vi "initalize 6221-2182-dc(SubVI).vi"(9 "字符串":string, 11 "簇":T13={"initialize"=enum."SR830", "6221"={"6221 Resource"="GPIB0::24::INSTR", "Delta status"=FALSE, "电流|RMS(A)"=0.0}, "SR830+6221"={"source"=0, "Current(A)"=0.0, "阻抗(Ohm)"=0.0, "SR830 1"=FALSE, "SR830 2"=FALSE, "SR830 3"=FALSE, "SR830 4"=FALSE, "VISA 1"="", "VISA 2"="", "VISA 3"="", "VISA 4"="", "Reserve 1"=0, "Reserve 2"=-1, "Reserve 3"=-1, "Reserve 4"=-1, "Sensitivity 1"=-1, "Sensitivity 2"=0, "Sensitivity 3"=-1, "Sensitivity 4"=-1, "量程入 1"=0, "量程入 2"=0, "量程入 3"=0, "量程入 4"=0}, "2400"={"2400"=FALSE, "VISA"="", "Output Level (0)"=1e-05, "Compliance  Level (0.1)"=10.0}, "ch"={"ch"=[], "current"=[], "change?"=[], "holding current\nwhen change ch?"=FALSE}, "Instrument"={"335 Resource"="GPIB0::24::INSTR", "Input (0:A)"=0, "Instrument Type"=enum."PPMS-Rotate", "quantum design"=refnum, "Heater Output (1:1)"=1, "semaphore"=refnum, "TCP master instance"=refnum, "335 Status"=refnum, "M24C Resource"="GPIB0::24::INSTR", "4G supply"="GPIB0::24::INSTR", "Temp Status 24C"=refnum, "Temp"=refnum, "9T信号"=refnum, "limit"={"Field limit"=0.0, "Field rate limit"=0.0, "Temp limit"=0.0, "Temp low limit"=0.0, "Temp rate limit "=0.0}, "4g supply status"=refnum, "vi路径"="", "325 Resource "="GPIB0::24::INSTR", "Input (0:A) 325"=0, "Input (1;B)"=1, "in-plane"="", "out-plane"="", "in-plane"=FALSE, "out-plane"=FALSE}, "Aborting"=refnum, "数据文件"=refnum, "warning"=refnum, "2614B"={"2614B chA"=FALSE, "2614B chB"=FALSE, "VISA"=""}, "33522b"={"33522b resource name"="", "零电压"=0.0, "最大电压"=148.0, "间隔"=4.0, "最小电压"=-48.0, "PZT Scan?"=FALSE}, "gating type"=enum."2614(daul)"} {"Instrument"."Input (1;B)" items=["A", "B"]; "Instrument"."Input (0:A) 325" items=["A", "B"]; "Instrument"."Input (0:A)" items=["A", "B"]; "Instrument"."Heater Output (1:1)" items=["1"=1, "2"=2]; "SR830+6221"."Sensitivity 4" items=["Auto Gain"=-1, "2 nV/fA"=0, "5 nV/fA"=1, "10 nV/fA"=2, "20 nV/fA"=3, "50 nV/fA"=4, "100 nV/fA"=5, "200 nV/fA"=6, "500 nV/fA"=7, "1 uV/pA"=8, "2 uV/pA"=9, "5 uV/pA"=10, "10 uV/pA"=11, "20 uV/pA"=12, "50 uV/pA"=13, "100 uV/pA"=14, "200 uV/pA"=15, "500 uV/pA"=16, "1 mV/nA"=17, "2 mV/nA"=18, "5 mV/nA"=19, "10 mV/nA"=20, "20 mV/nA"=21, "50 mV/nA"=22, "100 mV/nA"=23, "200 mV/nA"=24, "500 mV/mA"=25, "1 V/uA"=26]; "SR830+6221"."Sensitivity 3" items=["Auto Gain"=-1, "2 nV/fA"=0, "5 nV/fA"=1, "10 nV/fA"=2, "20 nV/fA"=3, "50 nV/fA"=4, "100 nV/fA"=5, "200 nV/fA"=6, "500 nV/fA"=7, "1 uV/pA"=8, "2 uV/pA"=9, "5 uV/pA"=10, "10 uV/pA"=11, "20 uV/pA"=12, "50 uV/pA"=13, "100 uV/pA"=14, "200 uV/pA"=15, "500 uV/pA"=16, "1 mV/nA"=17, "2 mV/nA"=18, "5 mV/nA"=19, "10 mV/nA"=20, "20 mV/nA"=21, "50 mV/nA"=22, "100 mV/nA"=23, "200 mV/nA"=24, "500 mV/mA"=25, "1 V/uA"=26]; "SR830+6221"."Sensitivity 1" items=["Auto Gain"=-1, "2 nV/fA"=0, "5 nV/fA"=1, "10 nV/fA"=2, "20 nV/fA"=3, "50 nV/fA"=4, "100 nV/fA"=5, "200 nV/fA"=6, "500 nV/fA"=7, "1 uV/pA"=8, "2 uV/pA"=9, "5 uV/pA"=10, "10 uV/pA"=11, "20 uV/pA"=12, "50 uV/pA"=13, "100 uV/pA"=14, "200 uV/pA"=15, "500 uV/pA"=16, "1 mV/nA"=17, "2 mV/nA"=18, "5 mV/nA"=19, "10 mV/nA"=20, "20 mV/nA"=21, "50 mV/nA"=22, "100 mV/nA"=23, "200 mV/nA"=24, "500 mV/mA"=25, "1 V/uA"=26]; "SR830+6221"."Sensitivity 2" items=["Auto Gain"=-1, "2 nV/fA"=0, "5 nV/fA"=1, "10 nV/fA"=2, "20 nV/fA"=3, "50 nV/fA"=4, "100 nV/fA"=5, "200 nV/fA"=6, "500 nV/fA"=7, "1 uV/pA"=8, "2 uV/pA"=9, "5 uV/pA"=10, "10 uV/pA"=11, "20 uV/pA"=12, "50 uV/pA"=13, "100 uV/pA"=14, "200 uV/pA"=15, "500 uV/pA"=16, "1 mV/nA"=17, "2 mV/nA"=18, "5 mV/nA"=19, "10 mV/nA"=20, "20 mV/nA"=21, "50 mV/nA"=22, "100 mV/nA"=23, "200 mV/nA"=24, "500 mV/mA"=25, "1 V/uA"=26]; "SR830+6221"."Reserve 4" items=["Auto Gain"=-1, "2 nV/fA"=0, "5 nV/fA"=1, "10 nV/fA"=2, "20 nV/fA"=3, "50 nV/fA"=4, "100 nV/fA"=5, "200 nV/fA"=6, "500 nV/fA"=7, "1 uV/pA"=8, "2 uV/pA"=9, "5 uV/pA"=10, "10 uV/pA"=11, "20 uV/pA"=12, "50 uV/pA"=13, "100 uV/pA"=14, "200 uV/pA"=15, "500 uV/pA"=16, "1 mV/nA"=17, "2 mV/nA"=18, "5 mV/nA"=19, "10 mV/nA"=20, "20 mV/nA"=21, "50 mV/nA"=22, "100 mV/nA"=23, "200 mV/nA"=24, "500 mV/mA"=25, "1 V/uA"=26]; "SR830+6221"."Reserve 3" items=["Auto Reserve"=-1, "High Reserve"=0, "Normal"=1, "Low Noise"=2]; "SR830+6221"."Reserve 2" items=["Auto Reserve"=-1, "High Reserve"=0, "Normal"=1, "Low Noise"=2]; "SR830+6221"."Reserve 1" items=["Auto Reserve"=-1, "High Reserve"=0, "Normal"=1, "Low Noise"=2]; "SR830+6221"."source" items=["SR830 1", "SR830 2", "SR830 3", "SR830 4"]}) -> (3 "输出簇":T13={"initialize"=enum."SR830", "6221"={"6221 Resource"="GPIB0::24::INSTR", "Delta status"=FALSE, "电流|RMS(A)"=0.0}, "SR830+6221"={"source"=0, "Current(A)"=0.0, "阻抗(Ohm)"=0.0, "SR830 1"=FALSE, "SR830 2"=FALSE, "SR830 3"=FALSE, "SR830 4"=FALSE, "VISA 1"="", "VISA 2"="", "VISA 3"="", "VISA 4"="", "Reserve 1"=0, "Reserve 2"=-1, "Reserve 3"=-1, "Reserve 4"=-1, "Sensitivity 1"=-1, "Sensitivity 2"=0, "Sensitivity 3"=-1, "Sensitivity 4"=-1, "量程入 1"=0, "量程入 2"=0, "量程入 3"=0, "量程入 4"=0}, "2400"={"2400"=FALSE, "VISA"="", "Output Level (0)"=1e-05, "Compliance  Level (0.1)"=10.0}, "ch"={"ch"=[], "current"=[], "change?"=[], "holding current\nwhen change ch?"=FALSE}, "Instrument"={"335 Resource"="GPIB0::24::INSTR", "Input (0:A)"=0, "Instrument Type"=enum."PPMS-Rotate", "quantum design"=refnum, "Heater Output (1:1)"=1, "semaphore"=refnum, "TCP master instance"=refnum, "335 Status"=refnum, "M24C Resource"="GPIB0::24::INSTR", "4G supply"="GPIB0::24::INSTR", "Temp Status 24C"=refnum, "Temp"=refnum, "9T信号"=refnum, "limit"={"Field limit"=0.0, "Field rate limit"=0.0, "Temp limit"=0.0, "Temp low limit"=0.0, "Temp rate limit "=0.0}, "4g supply status"=refnum, "vi路径"="", "325 Resource "="GPIB0::24::INSTR", "Input (0:A) 325"=0, "Input (1;B)"=1, "in-plane"="", "out-plane"="", "in-plane"=FALSE, "out-plane"=FALSE}, "Aborting"=refnum, "数据文件"=refnum, "warning"=refnum, "2614B"={"2614B chA"=FALSE, "2614B chB"=FALSE, "VISA"=""}, "33522b"={"33522b resource name"="", "零电压"=0.0, "最大电压"=148.0, "间隔"=4.0, "最小电压"=-48.0, "PZT Scan?"=FALSE}, "gating type"=enum."2614(daul)"} {"Instrument"."Input (1;B)" items=["A", "B"]; "Instrument"."Input (0:A) 325" items=["A", "B"]; "Instrument"."Input (0:A)" items=["A", "B"]; "Instrument"."Heater Output (1:1)" items=["1"=1, "2"=2]; "SR830+6221"."Sensitivity 4" items=["Auto Gain"=-1, "2 nV/fA"=0, "5 nV/fA"=1, "10 nV/fA"=2, "20 nV/fA"=3, "50 nV/fA"=4, "100 nV/fA"=5, "200 nV/fA"=6, "500 nV/fA"=7, "1 uV/pA"=8, "2 uV/pA"=9, "5 uV/pA"=10, "10 uV/pA"=11, "20 uV/pA"=12, "50 uV/pA"=13, "100 uV/pA"=14, "200 uV/pA"=15, "500 uV/pA"=16, "1 mV/nA"=17, "2 mV/nA"=18, "5 mV/nA"=19, "10 mV/nA"=20, "20 mV/nA"=21, "50 mV/nA"=22, "100 mV/nA"=23, "200 mV/nA"=24, "500 mV/mA"=25, "1 V/uA"=26]; "SR830+6221"."Sensitivity 3" items=["Auto Gain"=-1, "2 nV/fA"=0, "5 nV/fA"=1, "10 nV/fA"=2, "20 nV/fA"=3, "50 nV/fA"=4, "100 nV/fA"=5, "200 nV/fA"=6, "500 nV/fA"=7, "1 uV/pA"=8, "2 uV/pA"=9, "5 uV/pA"=10, "10 uV/pA"=11, "20 uV/pA"=12, "50 uV/pA"=13, "100 uV/pA"=14, "200 uV/pA"=15, "500 uV/pA"=16, "1 mV/nA"=17, "2 mV/nA"=18, "5 mV/nA"=19, "10 mV/nA"=20, "20 mV/nA"=21, "50 mV/nA"=22, "100 mV/nA"=23, "200 mV/nA"=24, "500 mV/mA"=25, "1 V/uA"=26]; "SR830+6221"."Sensitivity 1" items=["Auto Gain"=-1, "2 nV/fA"=0, "5 nV/fA"=1, "10 nV/fA"=2, "20 nV/fA"=3, "50 nV/fA"=4, "100 nV/fA"=5, "200 nV/fA"=6, "500 nV/fA"=7, "1 uV/pA"=8, "2 uV/pA"=9, "5 uV/pA"=10, "10 uV/pA"=11, "20 uV/pA"=12, "50 uV/pA"=13, "100 uV/pA"=14, "200 uV/pA"=15, "500 uV/pA"=16, "1 mV/nA"=17, "2 mV/nA"=18, "5 mV/nA"=19, "10 mV/nA"=20, "20 mV/nA"=21, "50 mV/nA"=22, "100 mV/nA"=23, "200 mV/nA"=24, "500 mV/mA"=25, "1 V/uA"=26]; "SR830+6221"."Sensitivity 2" items=["Auto Gain"=-1, "2 nV/fA"=0, "5 nV/fA"=1, "10 nV/fA"=2, "20 nV/fA"=3, "50 nV/fA"=4, "100 nV/fA"=5, "200 nV/fA"=6, "500 nV/fA"=7, "1 uV/pA"=8, "2 uV/pA"=9, "5 uV/pA"=10, "10 uV/pA"=11, "20 uV/pA"=12, "50 uV/pA"=13, "100 uV/pA"=14, "200 uV/pA"=15, "500 uV/pA"=16, "1 mV/nA"=17, "2 mV/nA"=18, "5 mV/nA"=19, "10 mV/nA"=20, "20 mV/nA"=21, "50 mV/nA"=22, "100 mV/nA"=23, "200 mV/nA"=24, "500 mV/mA"=25, "1 V/uA"=26]; "SR830+6221"."Reserve 4" items=["Auto Gain"=-1, "2 nV/fA"=0, "5 nV/fA"=1, "10 nV/fA"=2, "20 nV/fA"=3, "50 nV/fA"=4, "100 nV/fA"=5, "200 nV/fA"=6, "500 nV/fA"=7, "1 uV/pA"=8, "2 uV/pA"=9, "5 uV/pA"=10, "10 uV/pA"=11, "20 uV/pA"=12, "50 uV/pA"=13, "100 uV/pA"=14, "200 uV/pA"=15, "500 uV/pA"=16, "1 mV/nA"=17, "2 mV/nA"=18, "5 mV/nA"=19, "10 mV/nA"=20, "20 mV/nA"=21, "50 mV/nA"=22, "100 mV/nA"=23, "200 mV/nA"=24, "500 mV/mA"=25, "1 V/uA"=26]; "SR830+6221"."Reserve 3" items=["Auto Reserve"=-1, "High Reserve"=0, "Normal"=1, "Low Noise"=2]; "SR830+6221"."Reserve 2" items=["Auto Reserve"=-1, "High Reserve"=0, "Normal"=1, "Low Noise"=2]; "SR830+6221"."Reserve 1" items=["Auto Reserve"=-1, "High Reserve"=0, "Normal"=1, "Low Noise"=2]; "SR830+6221"."source" items=["SR830 1", "SR830 2", "SR830 3", "SR830 4"]})   [LabVIEW 2019, in "initialize.lvlib"]
uses:
  initialize.lvlib
  ctl/config.ctl
  <vilib>/NI/Modbus Library/API/Master/Modbus Master.lvclass
  ctl/initialize.ctl
  ctl/Instrument.ctl
  ctl/Instrument Type.ctl
  lib/QDInstrument.dll
  ctl/335 state.ctl
  ctl/limit.ctl
  ctl/9T mag field stauts.ctl
  ctl/warning.ctl
  ctl/Gating type.ctl
  lib/Keithley 622x/Configure/Source/Typedefs/KE622x -- Current Range.ctl
  lib/Keithley 622x/Configure/Source/Typedefs/KE622x -- Current Ranges.ctl
  lib/Keithley 622x/Typedefs/KE622x -- On Off Control.ctl
  lib/Keithley 622x/Configure/Output/Typedefs/KE6221 -- Output Response.ctl
  lib/Keithley 622x/Configure/Source/Typedefs/KE622x -- Current Level.ctl
  lib/Keithley 622x/Configure/Source/Typedefs/KE622x -- Voltage Limit.ctl
  lib/Keithley 622x/Configure/2182 -A/Low Level/Typedefs/KE2182 -- Voltage Ranges.ctl
  lib/Keithley 622x/Configure/2182 -A/Low Level/Typedefs/KE2182 -- Filter Type.ctl
  lib/Keithley 622x/Configure/2182 -A/Low Level/Typedefs/KE2182 -- Filter Count.ctl
  lib/Keithley 622x/Configure/2182 -A/Low Level/Typedefs/KE2182 -- Filter Window.ctl
  lib/Keithley 622x/Configure/2182 -A/Low Level/Typedefs/KE2182 -- NPLCs.ctl
  lib/Keithley 622x/Utility/Typedefs/KE622x -- Instrument Type.ctl
  lib/Keithley 622x/Keithley 622x.lvlib
panel:
  in  "2812 -A Params In":T6={"Auto Range?"=FALSE, "Man / Selected\nRange"=enum."10mV", "Enable Digital\nFilter?"=FALSE, "Filter Type"=enum."Moving", "Filter Count"=10, "Filter\nWindow (%)"=0.01, "Enable Analog\nFilter?"=FALSE, "NPLCs"=5} {"Filter\nWindow (%)" min=0.0 max=10.0 step=0.01 format="%.2f"; "Filter Count" min=1 max=100; "NPLCs" min=1 max=10}
  in  "Turn Off Output If Voltage Limit?":bool=TRUE
  out "error out":errorcluster
  out "Voltage Limit?":bool
  out "Interlock Tripped?":bool
  in  "Voltage Limit (V)":T7=10.0 min=0.1 max=105.0 step=0.01 format="%.2p"
  in  "Current Level (A)":T8=0.001 min=-0.105 max=0.105 format="%.4p"
  in  "Output Response":T9=enum."Slow"
  in  "Analog Filter State":T10
  in  "Current Range In":T11={"Auto Range?"=TRUE, "Man / Selected\nRange"=enum."2nA"}
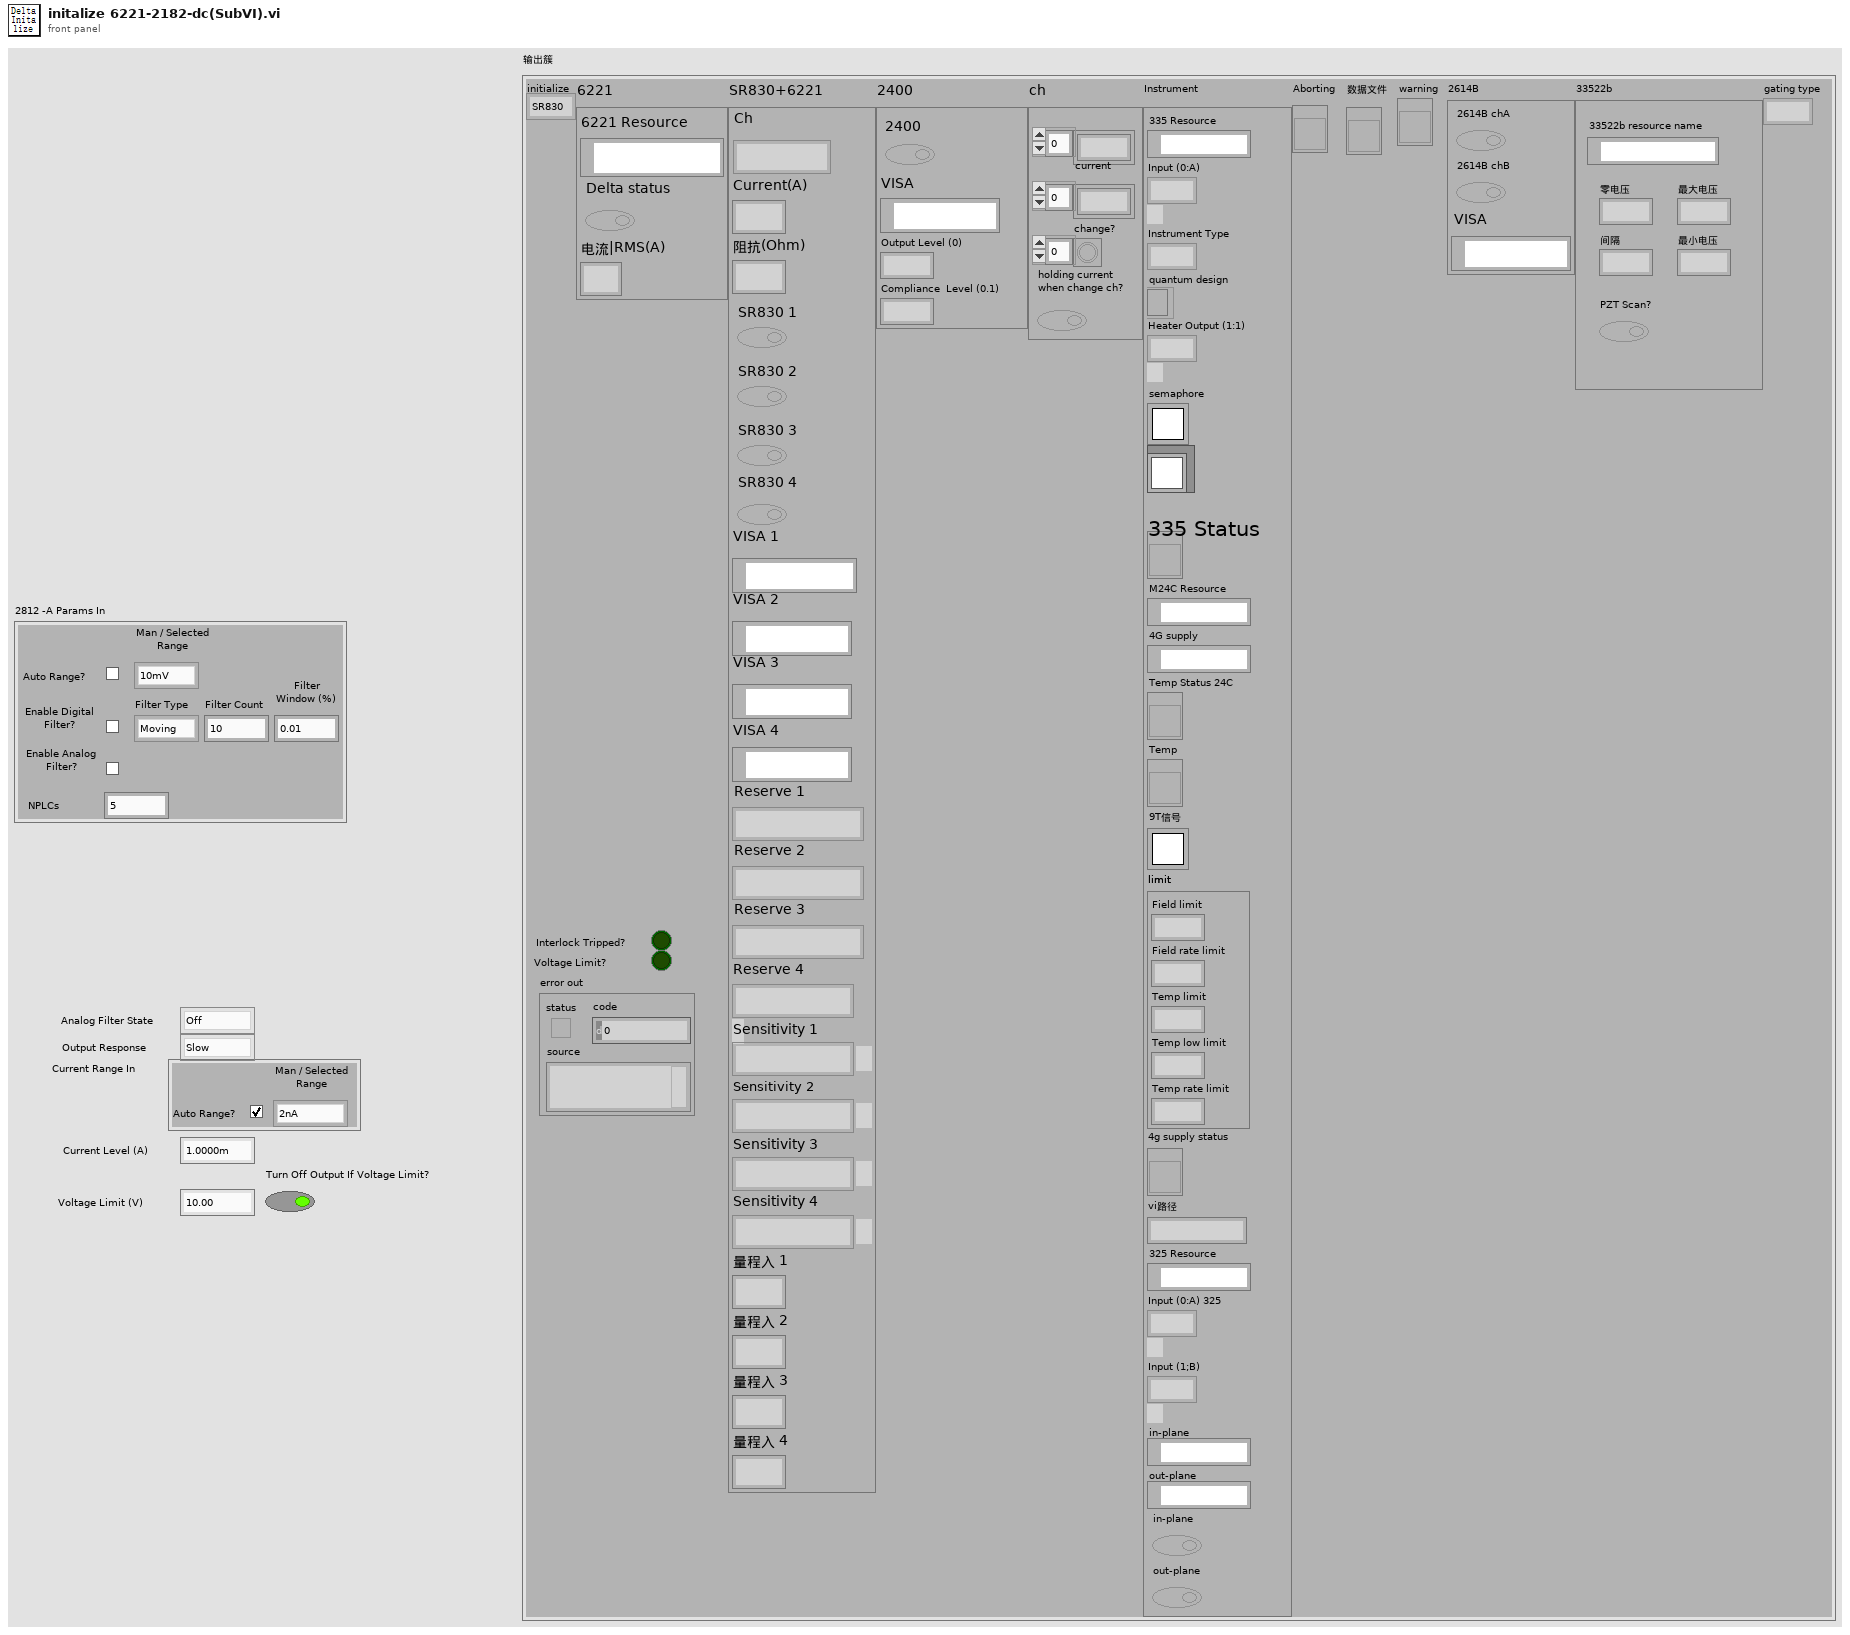
[diagram p1: front panel]
types:
  T1 = typedef "Keithley 622x.lvlib/KE2182 -- Voltage Ranges.ctl" = enum16{"10mV", "100mV", "1V", "10V", "100V"}
  T2 = typedef "Keithley 622x.lvlib/KE2182 -- Filter Type.ctl" = enum16{"Moving", "Repeat"}
  T3 = typedef "Keithley 622x.lvlib/KE2182 -- Filter Count.ctl" = u32
  T4 = typedef "Keithley 622x.lvlib/KE2182 -- Filter Window.ctl" = dbl
  T5 = typedef "Keithley 622x.lvlib/KE2182 -- NPLCs.ctl" = u32
  T6 = cluster{"Auto Range?":bool, "Man / Selected\nRange":T1, "Enable Digital\nFilter?":bool, "Filter Type":T2, "Filter Count":T3, "Filter\nWindow (%)":T4, "Enable Analog\nFilter?":bool, "NPLCs":T5}
  T7 = typedef "Keithley 622x.lvlib/KE622x -- Voltage Limit.ctl" = dbl
  T8 = typedef "Keithley 622x.lvlib/KE622x -- Current Level.ctl" = dbl
  T9 = typedef "Keithley 622x.lvlib/KE6221 -- Output Response.ctl" = enum16{"Fast", "Slow"}
  T10 = typedef "Keithley 622x.lvlib/KE622x -- On Off Control.ctl" = enum16{"Off", "On"}
  T11 = typedef "Keithley 622x.lvlib/KE622x -- Current Range.ctl" = cluster{"Auto Range?":bool, "Man / Selected\nRange":T12}
  T12 = typedef "Keithley 622x.lvlib/KE622x -- Current Ranges.ctl" = enum16{"2nA", "20nA", "200nA", "2uA", "20uA", "200uA", "2mA", "20mA", "100mA"}
  T13 = typedef "config.ctl" = cluster{"initialize":T14, "6221":cluster{"6221 Resource":refnum<visa-resource-name>, "Delta status":bool, "电流|RMS(A)":dbl}, "SR830+6221":cluster{"source":u16, "Current(A)":dbl, "阻抗(Ohm)":dbl, "SR830 1":bool, "SR830 2":bool, "SR830 3":bool, "SR830 4":bool, "VISA 1":refnum<visa-resource-name>, "VISA 2":refnum<visa-resource-name>, "VISA 3":refnum<visa-resource-name>, "VISA 4":refnum<visa-resource-name>, "Reserve 1":i16, "Reserve 2":i16, "Reserve 3":i16, "Reserve 4":i16, "Sensitivity 1":i16, "Sensitivity 2":i16, "Sensitivity 3":i16, "Sensitivity 4":i16, "量程入 1":i32, "量程入 2":i32, "量程入 3":i32, "量程入 4":i32}, "2400":cluster{"2400":bool, "VISA":refnum<visa-resource-name>, "Output Level (0)":dbl, "Compliance  Level (0.1)":dbl}, "ch":cluster{"ch":i32[], "current":dbl[], "change?":bool[], "holding current\nwhen change ch?":bool}, "Instrument":T15, "Aborting":refnum<vi>, "数据文件":refnum<vi>, "warning":refnum<vi>, "2614B":cluster{"2614B chA":bool, "2614B chB":bool, "VISA":refnum<visa-resource-name>}, "33522b":cluster{"33522b resource name":refnum<visa-resource-name>, "零电压":dbl, "最大电压":dbl, "间隔":dbl, "最小电压":dbl, "PZT Scan?":bool}, "gating type":T19}
  T14 = typedef "initialize.ctl" = enum16{"SR830", "keithley6221-SR830", "Delta", "Delta-tunnelling", "keithley6221-2182-DC", "PZT"}
  T15 = typedef "Instrument.ctl" = cluster{"335 Resource":refnum<visa-resource-name>, "Input (0:A)":u16, "Instrument Type":T16, "quantum design":refnum<k24>, "Heater Output (1:1)":u16, "semaphore":T17, "TCP master instance":refnum<class "Modbus Master.lvclass">, "335 Status":refnum<vi>, "M24C Resource":refnum<visa-resource-name>, "4G supply":refnum<visa-resource-name>, "Temp Status 24C":refnum<vi>, "Temp":refnum<vi>, "9T信号":T17, "limit":T18, "4g supply status":refnum<vi>, "vi路径":string, "325 Resource ":refnum<visa-resource-name>, "Input (0:A) 325":u16, "Input (1;B)":u16, "in-plane":refnum<visa-resource-name>, "out-plane":refnum<visa-resource-name>, "in-plane":bool, "out-plane":bool}
  T16 = typedef "Instrument Type.ctl" = enum16{"PPMS", "VersaLab", "DynaCool", "SVSM", "PPMS-Rotate", "Lakeshore335", "9T mag"}
  T17 = typedef "Semaphore RefNum" = refnum<k1>
  T18 = typedef "limit.ctl" = cluster{"Field limit":dbl, "Field rate limit":dbl, "Temp limit":dbl, "Temp low limit":dbl, "Temp rate limit ":dbl}
  T19 = typedef "Gating type.ctl" = enum32{"null", "2614(daul)", "2400"}
  T20 = typedef "Keithley 622x.lvlib/KE622x -- Instrument Type.ctl" = enum16{"KE6220", "KE6221"}
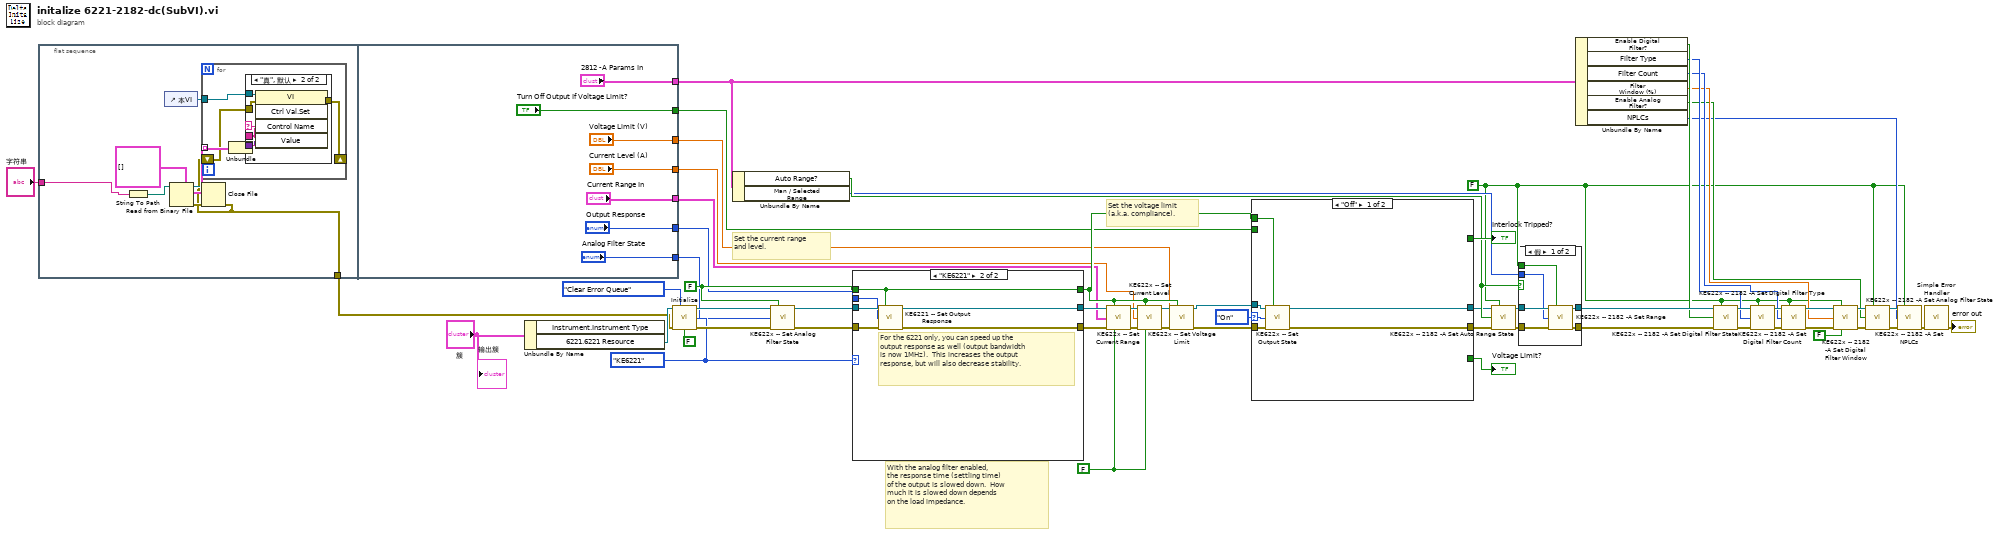
[diagram p0: block diagram]
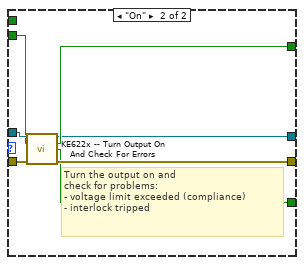
[diagram p3: hidden frame]
diagram:
  w9 = FALSE ("Check For SCPI Errors? (T)")
  w55 = KE622x_--_Instrument_Type."KE6221" ("Instrument Type")
  w53 = FALSE ("Check For SCPI Errors? (T)")
  w48 = FALSE ("Read Back Set Values? (T)")
  # "Set the voltage limit\n(a.k.a. compliance)."
  # "Set the current range\nand level."
  # "With the analog filter enabled,\nthe response time (settling time)\nof the output is slowed down.  How\nmuch it is slowed down depends\non the load impedance."
  n1 = flat-sequence {
    tunnel: "字符串" -> [w62]
    tunnel: [w61] -> w2
    tunnel: ["Current Range In"] -> w38
    tunnel: ["Analog Filter State"] -> w37
    tunnel: ["Output Response"] -> w36
    tunnel: ["Voltage Limit (V)"] -> w35
    tunnel: ["Current Level (A)"] -> w34
    tunnel: ["Turn Off Output If Voltage Limit?"] -> w33
    tunnel: ["2812 -A Params In"] -> w8
    frame #0 {
      n2 = String To Path(string=w62) -> (path=w67:path)
      n3 = control-ref of="本VI"() -> (w68:refnum<vi>)
      n4 = Read from Binary File(5:cluster{"Name":string, "Variant Data":variant}[] [] ("控件值:获取全部"), 11:w67) -> (0:w63:errorcluster, 2:w65:cluster{"Name":string, "Variant Data":variant}[], 3:w64:refnum<file>)  [unwired: 4 in, 1 out]
      n5 = Close File(refnum=w64, error in=w63) -> (error out=w61:errorcluster)  [unwired: 1 out]
      n6 = for {
        tunnel: w65 -> [w74] mode=indexing
        tunnel: w68 -> [w73]
        shift-right: [w69] -> _
        shift-left: w61 -> [w70]
        n7 = Unbundle(w74) -> ("Name"=w71:string, "Variant Data"=w72:variant)
        n8 = case shown="\"真\", 默认" w71 {
          tunnel: w73 -> [_ w80]
          tunnel: w71 -> [_ w79]
          tunnel: w72 -> [_ w78]
          tunnel: [w75 w77] -> w69
          tunnel: w70 -> [w75 w76]
          frame "cancel", "load", "model", "ok" {
          }
          frame "真", Default {
            n9 = invoke class="VI" method="Ctrl Val.Set"(reference=w80, error in=w76, "Control Name"=w79, "Value"=w78) -> (error out=w77:errorcluster)  [unwired: 1 in, 4 out]
          }
        }
      }
    }
    frame #1 {
    }
  }
  n10 = Unbundle By Name("簇") -> ("6221.6221 Resource"=w3:refnum<visa-resource-name>)  [unwired: 1 out]
  n11 = call "Initialize.vi"("VISA resource name"=w3, "Error Queue Option"=enum16{"Clear Error Queue", "Error Query"}."Clear Error Queue", "Instrument Type"=w55, "error in (no error)"=w2, "Reset? (T)"=FALSE) -> ("VISA resource name out"=w58:refnum<visa-resource-name>, "error out"=w57:errorcluster)  [unwired: 9 in]
  n12 = Unbundle By Name(w8) -> ("Auto Range?"=w18:bool, "Man / Selected\nRange"=w17:T1)
  n13 = call "KE622x -- Set Analog Filter State.vi"("Resource In"=w58, "Check For SCPI Errors? (T)"=w53, "Analog Filter State"=w37, "error in (no error)"=w57) -> ("Resource Out (dupl)"=w56:refnum<visa-resource-name>, "error out"=w54:errorcluster)  [unwired: 10 in]
  n14 = case shown="\"KE6221\"" w55 {
    tunnel: w56 -> [w89 w96]
    tunnel: w54 -> [w88 w95]
    tunnel: [w89 w94] -> w51
    tunnel: w53 -> [w90 w93]
    tunnel: [w90 w93] -> w41
    tunnel: [w88 w92] -> w52
    tunnel: w36 -> [_ w91]
    frame "KE6220" {
    }
    frame "KE6221" {
      # "For the 6221 only, you can speed up the\noutput response as well (output bandwidth\nis now 1MHz).  This increases the output\nresponse, but will also decrease stability."
      n15 = call "KE6221 -- Set Output Response.vi"("Resource In"=w96, "Check For SCPI Errors? (T)"=w93, "KE6221 Output Response"=w91, "error in (no error)"=w95) -> ("Resource Out (dupl)"=w94:refnum<visa-resource-name>, "error out"=w92:errorcluster)  [unwired: 10 in]
    }
  }
  n16 = call "KE622x -- Set Current Range.vi"("Resource In"=w51, "Check For SCPI Errors? (T)"=w41, "Current Range In"=w38, "error in (no error)"=w52, "Read Back Set Values? (T)"=w48) -> ("Resource Out (dupl)"=w50:refnum<visa-resource-name>, "error out"=w49:errorcluster)  [unwired: 8 in, 1 out]
  n17 = call "KE622x -- Set Current Level.vi"("Resource In"=w50, "Check For SCPI Errors? (T)"=w41, "Current Level (A) In"=w34, "error in (no error)"=w49, "Read Back Set Value? (T)"=w48) -> ("Resource Out (dupl)"=w47:refnum<visa-resource-name>, "error out"=w46:errorcluster)  [unwired: 8 in, 1 out]
  n18 = call "KE622x -- Set Voltage Limit.vi"("Resource In"=w47, "Check For SCPI Errors? (T)"=w41, "Voltage Limit (V)"=w35, "error in (no error)"=w46) -> ("Resource Out (dupl)"=w45:refnum<visa-resource-name>, "error out"=w44:errorcluster)  [unwired: 10 in]
  n19 = case shown="\"Off\"" KE622x_--_On_Off_Control."On" ("Output State") {
    selector: KE622x_--_On_Off_Control."On" ("Output State") -> [w100 _]
    tunnel: w45 -> [w102 w109]
    tunnel: w44 -> [w101 w108]
    tunnel: [w98 w107] -> w6
    tunnel: w41 -> [w99 _]
    tunnel: [_ w106] -> w40
    tunnel: [_ w105] -> w39
    tunnel: w33 -> [_ w104]
    tunnel: [w97 w103] -> w7
    frame "Off" {
      n20 = call "KE622x -- Set Output State.vi"("Resource In"=w102, "Check For SCPI Errors? (T)"=w99, "Output State"=w100, "error in (no error)"=w101) -> ("Resource Out (dupl)"=w97:refnum<visa-resource-name>, "error out"=w98:errorcluster)  [unwired: 10 in]
    }
    frame "On" {
      # "Turn the output on and\ncheck for problems:\n- voltage limit exceeded (compliance)\n- interlock tripped"
      n21 = call "KE622x -- Turn Output On And Check For Errors.vi"("Resource In"=w109, "Turn Off Output If Compliance?"=w104, "error in (no error)"=w108) -> ("Resource Out (dupl)"=w103:refnum<visa-resource-name>, "Interlock Tripped?"=w106:bool, "Compliance?"=w105:bool, "error out"=w107:errorcluster)  [unwired: 9 in]
    }
  }
  "Interlock Tripped?" <- w40
  "Voltage Limit?" <- w39
  n22 = call "KE622x -- 2182 -A Set Auto Range State.vi"("622x Resource In"=w7, "Check For SCPI Errors? (T)"=w9, "Enable Auto Range?"=w18, "error in (no error)"=w6) -> ("622x Resource Out (dupl)"=w32:refnum<visa-resource-name>, "error out"=w31:errorcluster)  [unwired: 10 in]
  n23 = case shown="假" w18 {
    tunnel: w32 -> [w115 w117]
    tunnel: w31 -> [w114 w116]
    tunnel: [w113 w117] -> w30
    tunnel: [w112 w116] -> w29
    tunnel: w17 -> [w110 _]
    tunnel: w9 -> [w111 _]
    frame False {
      n24 = call "KE622x -- 2182 -A Set Range.vi"("622x Resource In"=w115, "Check For SCPI Errors? (T)"=w111, "2182/2182A Range"=w110, "error in (no error)"=w114) -> ("622x Resource Out (dupl)"=w113:refnum<visa-resource-name>, "error out"=w112:errorcluster)  [unwired: 10 in]
    }
    frame True {
    }
  }
  n25 = Unbundle By Name(w8) -> ("Enable Digital\nFilter?"=w16:bool, "Filter Type"=w15:T2, "Filter Count"=w14:T3, "Filter\nWindow (%)"=w13:T4, "Enable Analog\nFilter?"=w12:bool, "NPLCs"=w11:T5)
  n26 = call "KE622x -- 2182 -A Set Digital Filter State.vi"("622x Resource In"=w30, "Check For SCPI Errors? (T)"=w9, "Enable Digital Filter?"=w16, "error in (no error)"=w29) -> ("622x Resource Out (dupl)"=w28:refnum<visa-resource-name>, "error out"=w27:errorcluster)  [unwired: 10 in]
  n27 = call "KE622x -- 2182 -A Set Digital Filter Type.vi"("622x Resource In"=w28, "Check For SCPI Errors? (T)"=w9, "Filter Type"=w15, "error in (no error)"=w27) -> ("622x Resource Out (dupl)"=w26:refnum<visa-resource-name>, "error out"=w25:errorcluster)  [unwired: 10 in]
  n28 = call "KE622x -- 2182 -A Set Digital Filter Count.vi"("622x Resource In"=w26, "Check For SCPI Errors? (T)"=w9, "Filter Count"=w14, "error in (no error)"=w25) -> ("622x Resource Out (dupl)"=w21:refnum<visa-resource-name>, "error out"=w24:errorcluster)  [unwired: 10 in]
  n29 = call "KE622x -- 2182 -A Set Digital Filter Window.vi"("622x Resource In"=w21, "Check For SCPI Errors? (T)"=w9, "Filter Window In (%)"=w13, "error in (no error)"=w24, "Read Back Set Value? (T)"=FALSE) -> ("622x Resource Out (dupl)"=w20:refnum<visa-resource-name>, "error out"=w23:errorcluster)  [unwired: 9 in]
  n30 = call "KE622x -- 2182 -A Set Analog Filter State.vi"("622x Resource In"=w20, "Check For SCPI Errors? (T)"=w9, "Enable Analog Filter?"=w12, "error in (no error)"=w23) -> ("622x Resource Out (dupl)"=w19:refnum<visa-resource-name>, "error out"=w22:errorcluster)  [unwired: 10 in]
  n31 = call "KE622x -- 2182 -A Set NPLCs.vi"("622x Resource In"=w19, "Check For SCPI Errors? (T)"=w9, "2182 -A NPLCs"=w11, "error in (no error)"=w22) -> ("error out"=w5:errorcluster)  [unwired: 10 in, 1 out]
  n32 = call <vilib>:"Simple Error Handler.vi"("error in (no error)"=w5) -> ("error out"=→"error out":errorcluster)  [unwired: 4 in, 4 out]
  "输出簇" <- "簇"
